vi "Task8.vi"() -> ()   [LabVIEW 2017]
panel:
  out "Value:":string
  in  "Array":bool[](array[boolean])
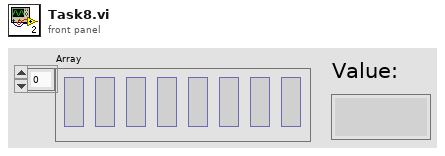
[diagram p1: front panel]
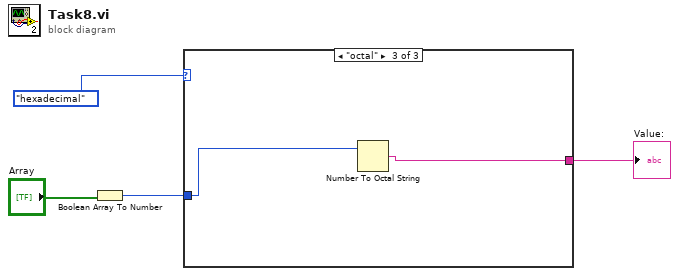
[diagram p0: block diagram]
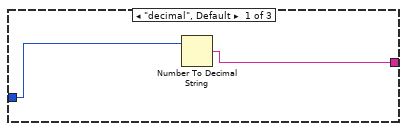
[diagram p2: hidden frame]
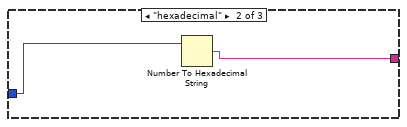
[diagram p3: hidden frame]
diagram:
  n1 = Boolean Array To Number(Boolean array="Array") -> (number=w2:u32)
  n2 = case shown="\"octal\"" enum8{"decimal", "octal", "hexadecimal"}."hexadecimal" {
    tunnel: w2 -> [w6 w8 w10]
    tunnel: [w5 w7 w9] -> w1
    frame "decimal", Default {
      n3 = Number To Decimal String(number=w6) -> (decimal integer string=w5:string)  [unwired: 1 in]
    }
    frame "hexadecimal" {
      n4 = Number To Hexadecimal String(2:w8) -> (0:w7:string)  [unwired: 1 in]
    }
    frame "octal" {
      n5 = Number To Octal String(2:w10) -> (0:w9:string)  [unwired: 1 in]
    }
  }
  "Value:" <- w1
